vi "LogDBBoolChange.vi"(6 "current time":timestamp, 7 "db table name":string, 8 "error in":errorcluster, 9 "value":bool, 10 "shiftReg":bool, 11 "Refnum in":T1) -> (0 "error out":errorcluster, 2 "shiftReg":bool, 3 "Refnum out":T1)   [LabVIEW 2011]
uses:
  <vilib>/addons/database/Connection.llb/Conn ObjectReference.ctl
  <vilib>/addons/database/NI_Database_API.lvlib
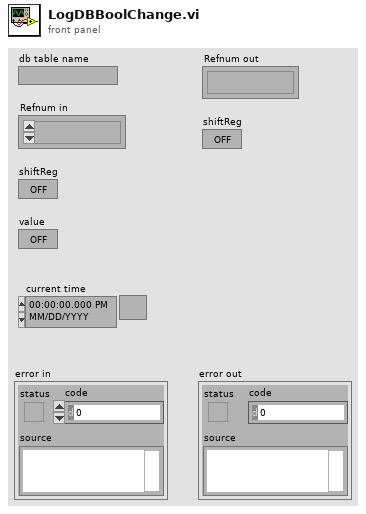
[diagram p1: front panel]
types:
  T1 = typedef "NI_Database_API.lvlib/Conn ObjectReference.ctl" = refnum<k1>
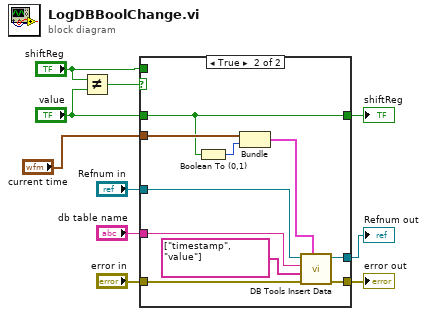
[diagram p0: block diagram]
diagram:
  n1 = Not Equal?(x="shiftReg", y="value") -> (x != y?=w4:bool)
  n2 = case shown="True" w4 {
    tunnel: [w11 w14] -> w8
    tunnel: [w13 w21] -> w7
    tunnel: "Refnum in" -> [w13 w22]
    tunnel: "db table name" -> [_ w23]
    tunnel: "error in" -> [w12 w20]
    tunnel: [w12 w19] -> w10
    tunnel: "current time" -> [_ w18]
    tunnel: "value" -> [_ w14]
    tunnel: "shiftReg" -> [w11 _]
    frame False {
    }
    frame True {
      n3 = Boolean To (0,1)(Boolean=w14) -> (0, 1=w15:i16)
      n4 = Bundle("current time"=w18, w15) -> (w17:cluster{"current time":timestamp, i16})  [unwired: 1 in]
      n5 = call <vilib>:"DB Tools Insert Data.vi"("data"=w17, "error in (no error)"=w20, "columns"=string[] ["timestamp", "value"], "table"=w23, "connection reference"=w22) -> ("error out"=w19:errorcluster, "connection reference out"=w21:T1)  [unwired: 5 in]
    }
  }
  "error out" <- w10
  "shiftReg" <- w8
  "Refnum out" <- w7
